vi "Gain OffsetLog.vi"(0 "Dynamic Data":dynamicdata(waveform)) -> (4 "Dynamic Data":dynamicdata(waveform))   [LabVIEW 2020]
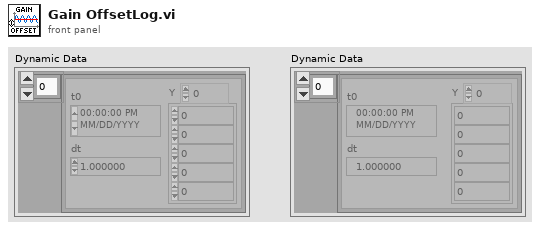
[diagram p1: front panel]
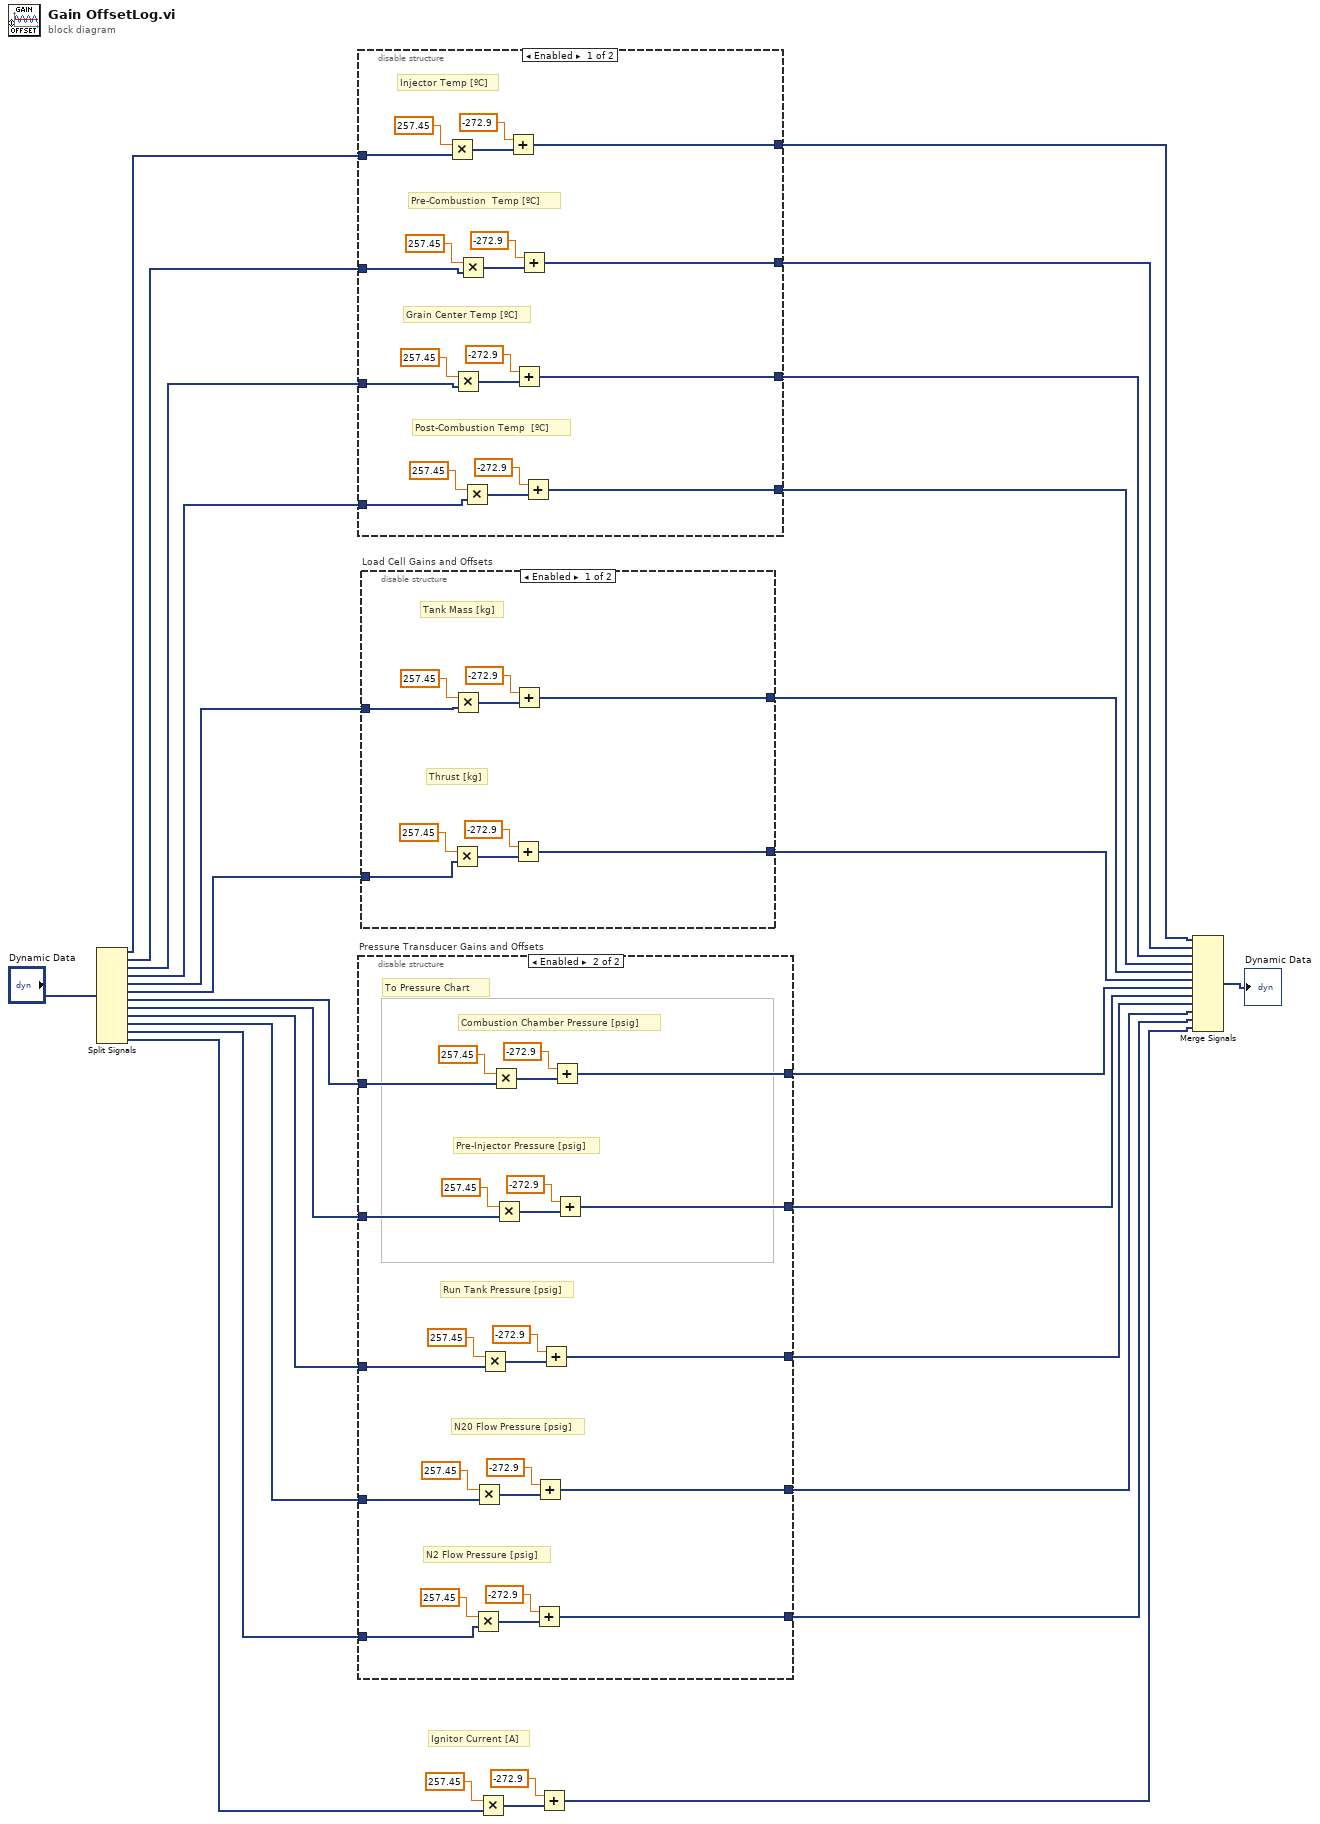
[diagram p0: block diagram]
diagram:
  # "Ignitor Current [A]"
  n1 = Split Signals("Dynamic Data") -> (w24:dynamicdata, w23:dynamicdata, w22:dynamicdata, w21:dynamicdata, w20:dynamicdata, w19:dynamicdata, w18:dynamicdata, w17:dynamicdata, w16:dynamicdata, w15:dynamicdata, w14:dynamicdata, w13:dynamicdata)  [unwired: 12 in]
  n2 = disable-structure shown="Enabled" {
    disable-tunnel: w24 -> [w37 _]
    disable-tunnel: w23 -> [w36 _]
    disable-tunnel: w22 -> [w35 _]
    disable-tunnel: w21 -> [w34 _]
    disable-tunnel: [w33 _] -> w12
    disable-tunnel: [w32 _] -> w11
    disable-tunnel: [w31 _] -> w10
    disable-tunnel: [w30 _] -> w9
    frame Enabled {
      # "Post-Combustion Temp  [ºC]"
      # "Grain Center Temp [ºC]"
      # "Pre-Combustion  Temp [ºC]"
      # "Injector Temp [ºC]"
      n3 = Multiply(x=257.45, y=w37) -> (x*y=w49:dynamicdata)
      n4 = Multiply(x=257.45, y=w35) -> (x*y=w43:dynamicdata)
      n5 = Multiply(x=257.45, y=w36) -> (x*y=w46:dynamicdata)
      n6 = Multiply(x=257.45, y=w34) -> (x*y=w40:dynamicdata)
      n7 = Add(x=-272.9, y=w49) -> (x+y=w33:dynamicdata)
      n8 = Add(x=-272.9, y=w43) -> (x+y=w31:dynamicdata)
      n9 = Add(x=-272.9, y=w46) -> (x+y=w32:dynamicdata)
      n10 = Add(x=-272.9, y=w40) -> (x+y=w30:dynamicdata)
    }
    frame Disabled {
    }
  }
  n11 = disable-structure "Pressure Transducer Gains and Offsets" shown="Enabled" {
    disable-tunnel: w18 -> [_ w59]
    disable-tunnel: w17 -> [_ w58]
    disable-tunnel: w16 -> [_ w57]
    disable-tunnel: w15 -> [_ w56]
    disable-tunnel: w14 -> [_ w55]
    disable-tunnel: [_ w54] -> w6
    disable-tunnel: [_ w53] -> w5
    disable-tunnel: [_ w52] -> w4
    disable-tunnel: [_ w51] -> w3
    disable-tunnel: [_ w50] -> w2
    frame Disabled {
    }
    frame Enabled {
      # "To Pressure Chart"
      # "Pre-Injector Pressure [psig]"
      # "N2 Flow Pressure [psig]"
      # "N20 Flow Pressure [psig]"
      # "Combustion Chamber Pressure [psig]"
      # "Run Tank Pressure [psig]"
      n12 = Multiply(x=257.45, y=w55) -> (x*y=w62:dynamicdata)
      n13 = Multiply(x=257.45, y=w56) -> (x*y=w65:dynamicdata)
      n14 = Multiply(x=257.45, y=w57) -> (x*y=w68:dynamicdata)
      n15 = Multiply(x=257.45, y=w59) -> (x*y=w74:dynamicdata)
      n16 = Multiply(x=257.45, y=w58) -> (x*y=w71:dynamicdata)
      n17 = Add(x=-272.9, y=w62) -> (x+y=w50:dynamicdata)
      n18 = Add(x=-272.9, y=w65) -> (x+y=w51:dynamicdata)
      n19 = Add(x=-272.9, y=w68) -> (x+y=w52:dynamicdata)
      n20 = Add(x=-272.9, y=w74) -> (x+y=w54:dynamicdata)
      n21 = Add(x=-272.9, y=w71) -> (x+y=w53:dynamicdata)
    }
  }
  n22 = disable-structure "Load Cell Gains and Offsets" shown="Enabled" {
    disable-tunnel: w20 -> [w78 _]
    disable-tunnel: w19 -> [w77 _]
    disable-tunnel: [w76 _] -> w8
    disable-tunnel: [w75 _] -> w7
    frame Enabled {
      # "Thrust [kg]"
      # "Tank Mass [kg]"
      n23 = Multiply(x=257.45, y=w77) -> (x*y=w81:dynamicdata)
      n24 = Multiply(x=257.45, y=w78) -> (x*y=w84:dynamicdata)
      n25 = Add(x=-272.9, y=w81) -> (x+y=w75:dynamicdata)
      n26 = Add(x=-272.9, y=w84) -> (x+y=w76:dynamicdata)
    }
    frame Disabled {
    }
  }
  n27 = Multiply(x=257.45, y=w13) -> (x*y=w27:dynamicdata)
  n28 = Add(x=-272.9, y=w27) -> (x+y=w1:dynamicdata)
  n29 = Merge Signals(w12, w11, w10, w9, w8, w7, w6, w5, w4, w3, w2, w1) -> (→"Dynamic Data":dynamicdata)
